vi "Get Valid data from string 2D array.vi"(11 "Value":string[][](array[string])) -> (1 "Cloumn Num":i32, 2 "Row Num":i32, 3 "Array":string[][](array[string]))   [LabVIEW 2021]
doc: "get the valid data number form string\n2016-03-21 10:26:33\n蒋松"
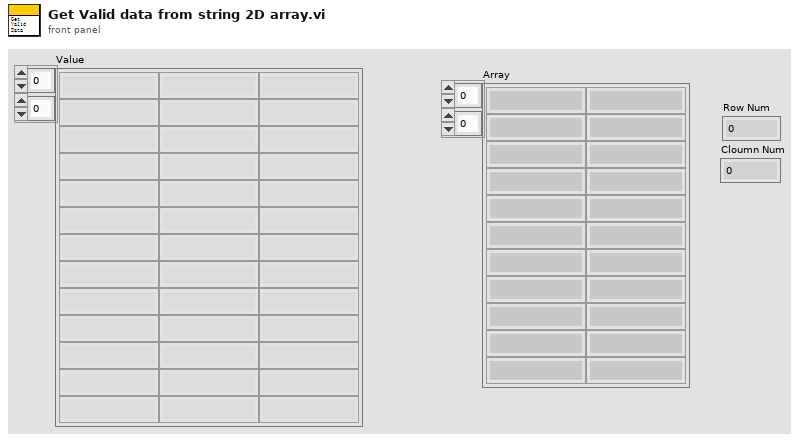
[diagram p1: front panel]
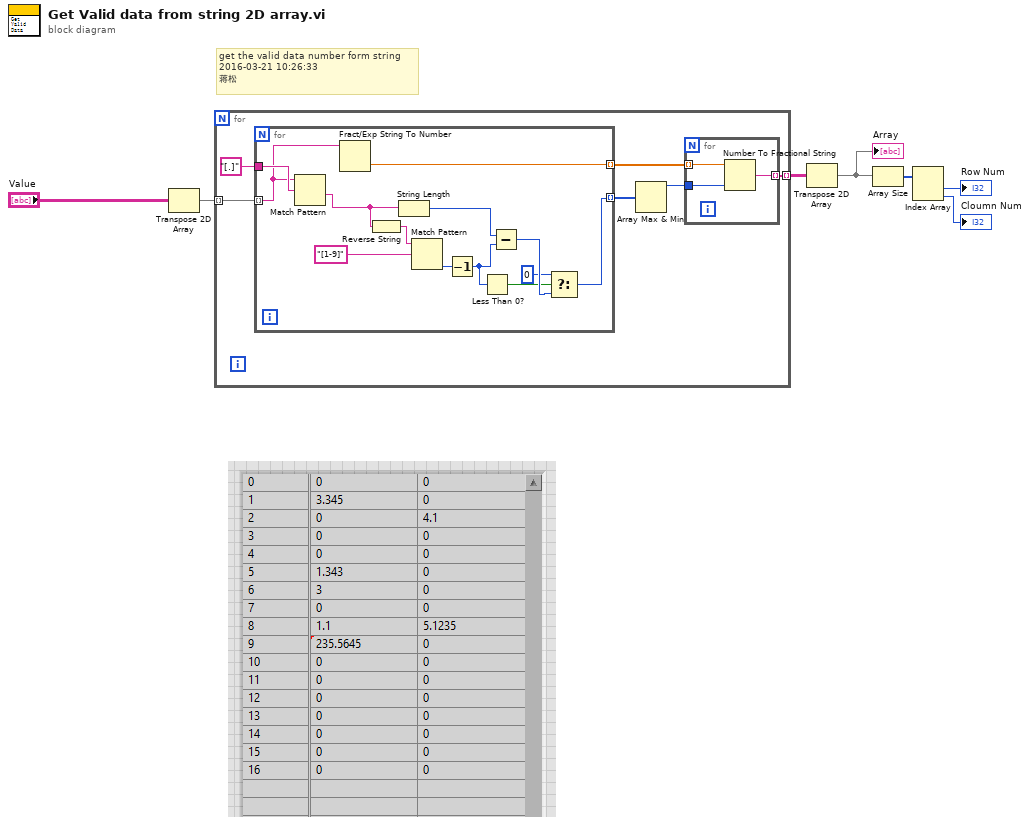
[diagram p0: block diagram]
diagram:
  # "get the valid data number form string\n2016-03-21 10:26:33\n蒋松"
  n1 = Transpose 2D Array(2D array="Value") -> (transposed array=w4:string[][])
  n2 = for {
    tunnel: w4 -> [w13] mode=indexing
    tunnel: [w8] -> w3 mode=indexing
    n3 = for {
      tunnel: w13 -> [w28] mode=indexing
      tunnel: [w17] -> w10 mode=indexing
      tunnel: "[.]" ("regular expression") -> [w29]
      tunnel: [w27] -> w9 mode=indexing
      n4 = Match Pattern(string=w28, regular expression=w29) -> (after substring=w18:string)  [unwired: 1 in, 3 out]
      n5 = Fract/Exp String To Number(string=w28) -> (number=w27:dbl)  [unwired: 3 in, 1 out]
      n6 = Reverse String(1:w18) -> (0:w20:string)
      n7 = String Length(string=w18) -> (length=w21:i32)
      n8 = Match Pattern(string=w20, regular expression="[1-9]") -> (offset past match=w22:i32)  [unwired: 1 in, 3 out]
      n9 = Decrement(x=w22) -> (x-1=w23:i32)
      n10 = Less Than 0?(x=w23) -> (x < 0?=w25:bool)
      n11 = Subtract(x=w21, y=w23) -> (x-y=w26:i32)
      n12 = Select(t=0, s=w25, f=w26) -> (s? t:f=w17:i32)
    }
    n13 = Array Max & Min(array=w10) -> (max value=w11:i32)  [unwired: 3 out]
    n14 = for {
      tunnel: w9 -> [w16] mode=indexing
      tunnel: w11 -> [w15]
      tunnel: [w14] -> w8 mode=indexing
      n15 = Number To Fractional String(number=w16, precision (6)=w15) -> (F-format string=w14:string)  [unwired: 2 in]
    }
  }
  n16 = Transpose 2D Array(2D array=w3) -> (transposed array=w1:string[][])
  "Array" <- w1
  n17 = Array Size(array=w1) -> (size(s)=w7:i32[])
  n18 = Index Array(array=w7) -> (element #1=→"Row Num":i32, element #2=→"Cloumn Num":i32)  [unwired: 2 in]
